vi "CreateSampleNameNode.vi"(8 "Error In":errorcluster, 10 "Sample":T1={"Name"="Sample Name", "Description"="Sample Description", "Molar Mass (g/mol)"=nan, "Density (g/cm^3)"=nan, "Irradiation Area (cm^2)"=nan, "SRIM Damage Peak (disp * ions/cm)"=nan}, 11 "DOM Document In":refnum<k20>) -> (0 "Error out":errorcluster, 2 "Sample Name Node":refnum<k20>, 3 "DOM Document Out":refnum<k20>)   [LabVIEW 2012]
uses:
  Sample.ctl
  <resource>/objmgr/DOMUserDefRef.rc
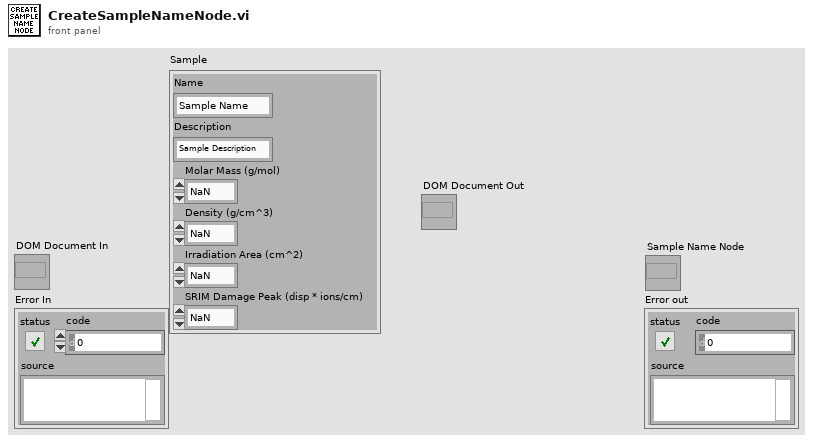
[diagram p1: front panel]
types:
  T1 = typedef "Sample.ctl" = cluster{"Name":string, "Description":string, "Molar Mass (g/mol)":dbl, "Density (g/cm^3)":dbl, "Irradiation Area (cm^2)":dbl, "SRIM Damage Peak (disp * ions/cm)":dbl}
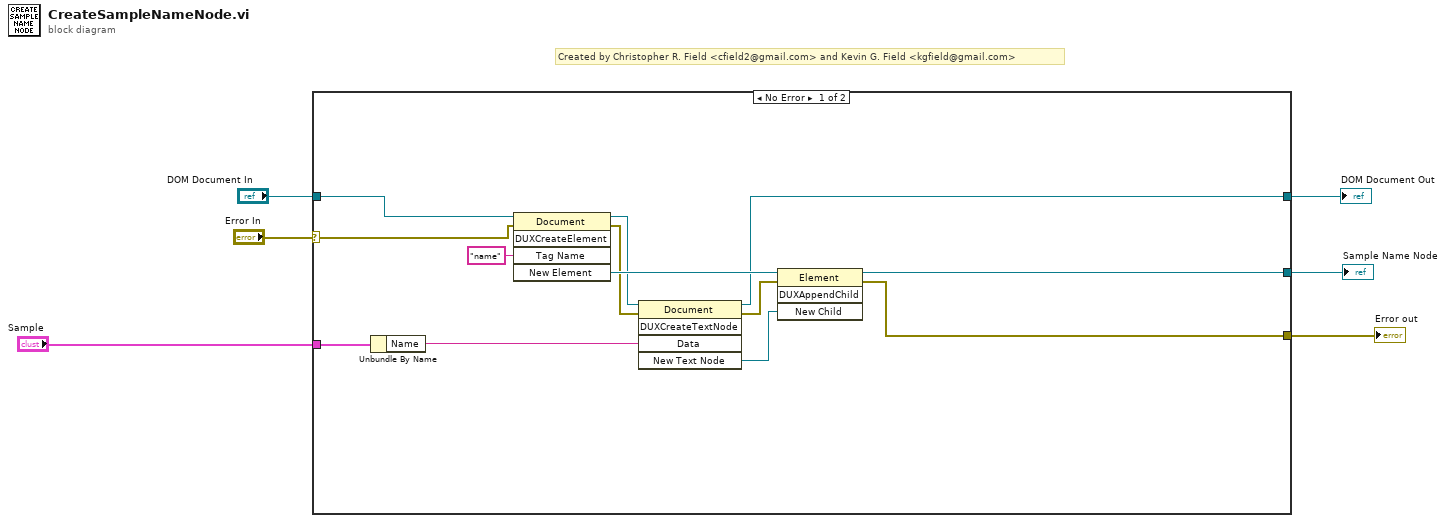
[diagram p0: block diagram]
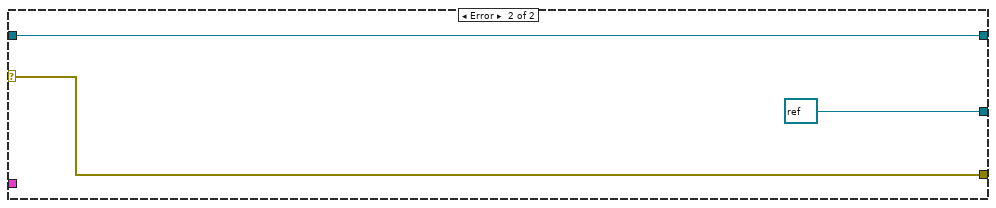
[diagram p2: hidden frame]
diagram:
  # "Created by Christopher R. Field <cfield2@gmail.com> and Kevin G. Field <kgfield@gmail.com>"
  n1 = case shown="No Error" "Error In" {
    selector: "Error In" -> [w9 w21]
    tunnel: "DOM Document In" -> [w19 w22]
    tunnel: [w18 refnum<k20> refnum ("Operator Node 2")] -> w5
    tunnel: [w17 w21] -> w4
    tunnel: "Sample" -> [w10 _]
    tunnel: [w8 w22] -> w2
    frame No Error {
      n2 = Unbundle By Name(w10) -> ("Name"=w7:string)
      n3 = invoke class="Document" method="DUXCreateElement"(reference=w19, error in=w9, "Tag Name"="name") -> (reference out=w14:refnum<k20>, error out=w13:errorcluster, "New Element"=w15:refnum<k20>)  [unwired: 2 in, 2 out]
      n4 = invoke class="Document" method="DUXCreateTextNode"(reference=w14, error in=w13, "Data"=w7) -> (reference out=w8:refnum<k20>, error out=w12:errorcluster, "New Text Node"=w11:refnum<k20>)  [unwired: 2 in, 2 out]
      n5 = invoke class="Element" method="DUXAppendChild"(reference=w15, error in=w12, "New Child"=w11) -> (reference out=w18:refnum<k20>, error out=w17:errorcluster)  [unwired: 1 in, 2 out]
    }
    frame Error {
    }
  }
  "Sample Name Node" <- w5
  "Error out" <- w4
  "DOM Document Out" <- w2
